vi "Find Latch Trip Reason.vi"(10 "FPGA Interface":T1) -> (1 "bBSPDDashLight":bool, 2 "bIMDDashLight":bool, 3 "bBMSDashLight":bool)   [LabVIEW 2015]
uses:
  FPGA Typedef.ctl
  <vilib>/rvi/errors/niLvFpgaAdjustHostInterfaceError.vi
  <vilib>/Utility/error.llb/Error Cluster From Error Code.vi
  <vilib>/rvi/interface/nirviReadWriteControl/nirviReadWriteControl.xnode
  FPGA Bitfiles/Latest.lvbitx
  NiFpgaLv.dll
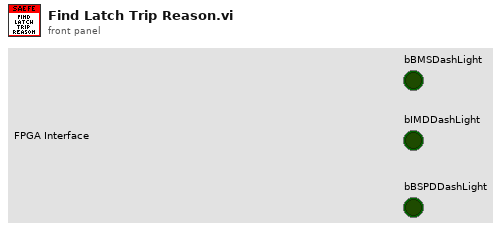
[diagram p1: front panel]
types:
  T1 = typedef "FPGA Typedef.ctl" = refnum<k20>
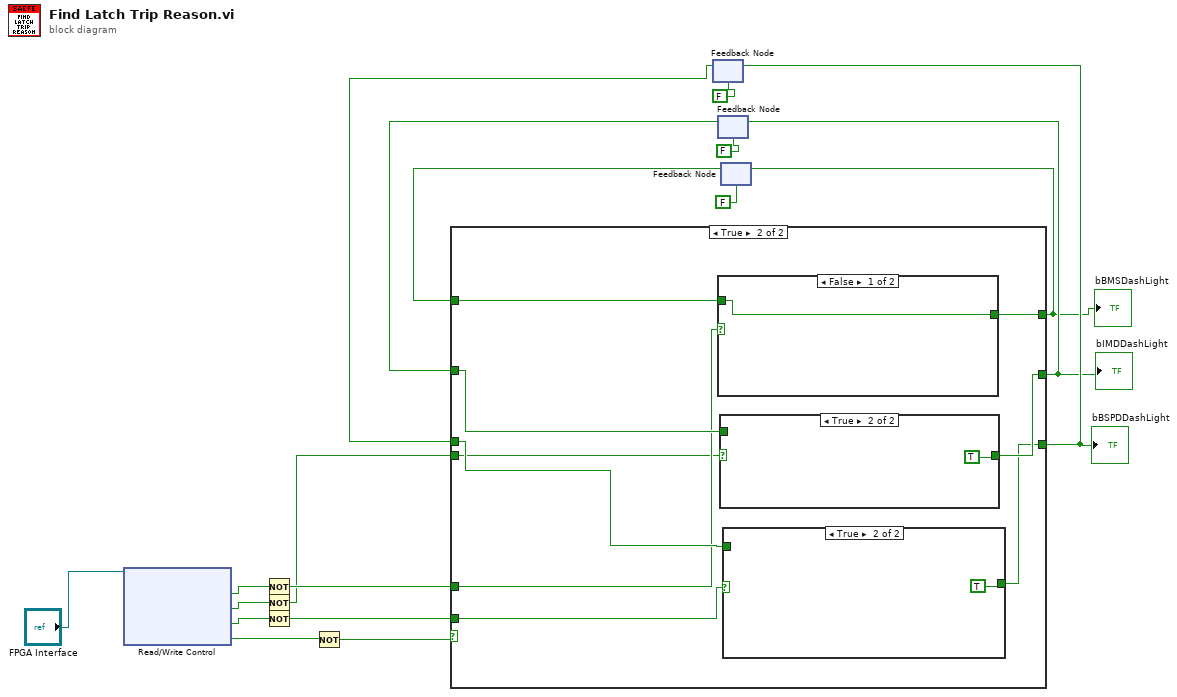
[diagram p0: block diagram]
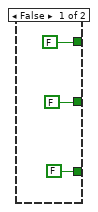
[diagram p2: hidden frame]
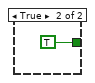
[diagram p5: hidden frame]
diagram:
  n1 = xnode "Read/Write Control"("FPGA VI Reference In"="FPGA Interface") -> ("bBMSOK"=w4:bool, "bIMDOK"=w3:bool, "bBSPDOK"=w2:bool, "bTSMSOutStatus"=w1:bool)  [unwired: 1 in, 2 out]
  n2 = Not(x=w4) -> (.not. x?=w9:bool)
  n3 = Not(x=w3) -> (.not. x?=w8:bool)
  n4 = Not(x=w2) -> (.not. x?=w7:bool)
  n5 = Not(x=w1) -> (.not. x?=w6:bool)
  n6 = feedback #1(FALSE) -> (w10:bool)
  n7 = feedback #2(FALSE) -> (w11:bool)
  n8 = feedback #3(FALSE) -> (w12:bool)
  n9 = case shown="True" w6 {
    tunnel: [FALSE w30] -> w13
    tunnel: [FALSE w29] -> w14
    tunnel: [FALSE w28] -> w15
    tunnel: w12 -> [_ w27]
    tunnel: w11 -> [_ w26]
    tunnel: w10 -> [_ w25]
    tunnel: w9 -> [_ w24]
    tunnel: w8 -> [_ w23]
    tunnel: w7 -> [_ w22]
    frame False {
    }
    frame True {
      n10 = case shown="False" w24 {
        tunnel: [w35 TRUE] -> w30
        tunnel: w27 -> [w35 _]
        frame False {
        }
        frame True {
        }
      }
      n11 = case shown="True" w23 {
        tunnel: [w33 TRUE] -> w29
        tunnel: w26 -> [w33 _]
        frame False {
        }
        frame True {
        }
      }
      n12 = case shown="True" w22 {
        tunnel: [w31 TRUE] -> w28
        tunnel: w25 -> [w31 _]
        frame False {
        }
        frame True {
        }
      }
    }
  }
  "bBMSDashLight" <- w13
  "bIMDDashLight" <- w14
  "bBSPDDashLight" <- w15
  n13 = feedback-in #1(w15) -> ()
  n14 = feedback-in #2(w14) -> ()
  n15 = feedback-in #3(w13) -> ()
